vi "Main.vi"(8 "Error In":errorcluster, 11 "Simulate hardware?":bool) -> (0 "Error Out":errorcluster={"status"=FALSE, "code"=1073676294, "source"="VISA Read in Monochromator.lvlib:ReadWrite.vi->Monochromator.lvlib:move.vi:1990001->Monochromator.lvlib:moveBothMonos.vi->Monochromator.lvlib:Main.vi"})   [LabVIEW 2017, in "Monochromator.lvlib"]
uses:
  Monochromator.lvlib
  Controls/Commands [enum].ctl
  Controls/Params.ctl
  Controls/Type.ctl
  Controls/GratingValues.ctl
  Controls/Grating.ctl
  PTI/Controls/Params.ctl
  Controls/VISA parameters.ctl
  Custom Oriel drivers/Controls/Params.ctl
  C:/Project Work/icl-optical-software-rewrite/Optical Software Code Simplified/Modules/Monochromator/Cornerstone.dll
  Cornerstone.dll
  Events/Controls/Action Refs [enum].ctl
  PTI/PTI.lvlib
  System Control/Main controller.lvlib
  Events/Events.lvlib
  File IO/File IO.lvlib
  Custom Oriel drivers/Oriel (custom drivers).lvlib
  Serial comms/Serial comms.lvlib
panel:
  out "Monochromator out":T1={"Type"=enum."PTI", "Wavelength (nm)"=600.0, "Grating, gr/mm"=enum."1200", "Grating mode"=enum."Unknown", "Spectrum mode"={"Spectrum mode?"=FALSE, "Start wavelength (nm)"=0.0, "End wavelength (nm)"=0.0, "Wavelength step (nm)"=0.0, "Wavelength array"=[], "array index"=0}, "PTI"={"Delay before read (ms)"=300, "Mono 1"={"Timeout (ms)"=1000, "Resource Name"="COM5", "Baud Rate"=9600, "Data Bits"=8, "Parity"=0, "Stop Bits"=10, "Flow Control"=0}, "Mono 2"={"Timeout (ms)"=1000, "Resource Name"="COM6", "Baud Rate"=9600, "Data Bits"=8, "Parity"=0, "Stop Bits"=10, "Flow Control"=0}, "Two PTI Monochromators?"=FALSE}, "Oriel (custom)"={"reference"=refnum}, "Force wavelength confirmation (PTI)?"=FALSE} {"PTI"."Mono 2"."Flow Control" items=["1.0"=10, "1.5"=15, "2.0"=20]; "PTI"."Mono 2"."Stop Bits" items=["None", "Odd", "Even", "Mark", "Space"]; "PTI"."Mono 2"."Parity" items=["None", "Odd", "Even", "Mark", "Space"]; "PTI"."Mono 1"."Flow Control" items=["1.0"=10, "1.5"=15, "2.0"=20]; "PTI"."Mono 1"."Stop Bits" items=["None", "Odd", "Even", "Mark", "Space"]; "PTI"."Mono 1"."Parity" items=["None", "Odd", "Even", "Mark", "Space"]}
  out "Test":bool=TRUE
  in  "Monochromator":T1={"Type"=enum."PTI", "Wavelength (nm)"=600.0, "Grating, gr/mm"=enum."1200", "Grating mode"=enum."Unknown", "Spectrum mode"={"Spectrum mode?"=FALSE, "Start wavelength (nm)"=0.0, "End wavelength (nm)"=0.0, "Wavelength step (nm)"=0.0, "Wavelength array"=[], "array index"=0}, "PTI"={"Delay before read (ms)"=300, "Mono 1"={"Timeout (ms)"=1000, "Resource Name"="COM5", "Baud Rate"=9600, "Data Bits"=8, "Parity"=0, "Stop Bits"=10, "Flow Control"=0}, "Mono 2"={"Timeout (ms)"=1000, "Resource Name"="COM6", "Baud Rate"=9600, "Data Bits"=8, "Parity"=0, "Stop Bits"=10, "Flow Control"=0}, "Two PTI Monochromators?"=FALSE}, "Oriel (custom)"={"reference"=refnum}, "Force wavelength confirmation (PTI)?"=TRUE} {"PTI"."Mono 2"."Flow Control" items=["1.0"=10, "1.5"=15, "2.0"=20]; "PTI"."Mono 2"."Stop Bits" items=["None", "Odd", "Even", "Mark", "Space"]; "PTI"."Mono 2"."Parity" items=["None", "Odd", "Even", "Mark", "Space"]; "PTI"."Mono 1"."Flow Control" items=["1.0"=10, "1.5"=15, "2.0"=20]; "PTI"."Mono 1"."Stop Bits" items=["None", "Odd", "Even", "Mark", "Space"]; "PTI"."Mono 1"."Parity" items=["None", "Odd", "Even", "Mark", "Space"]}
  in  "Stop Button":bool
  in  "move to wavelength":dbl=200.0
  in  "State":T8
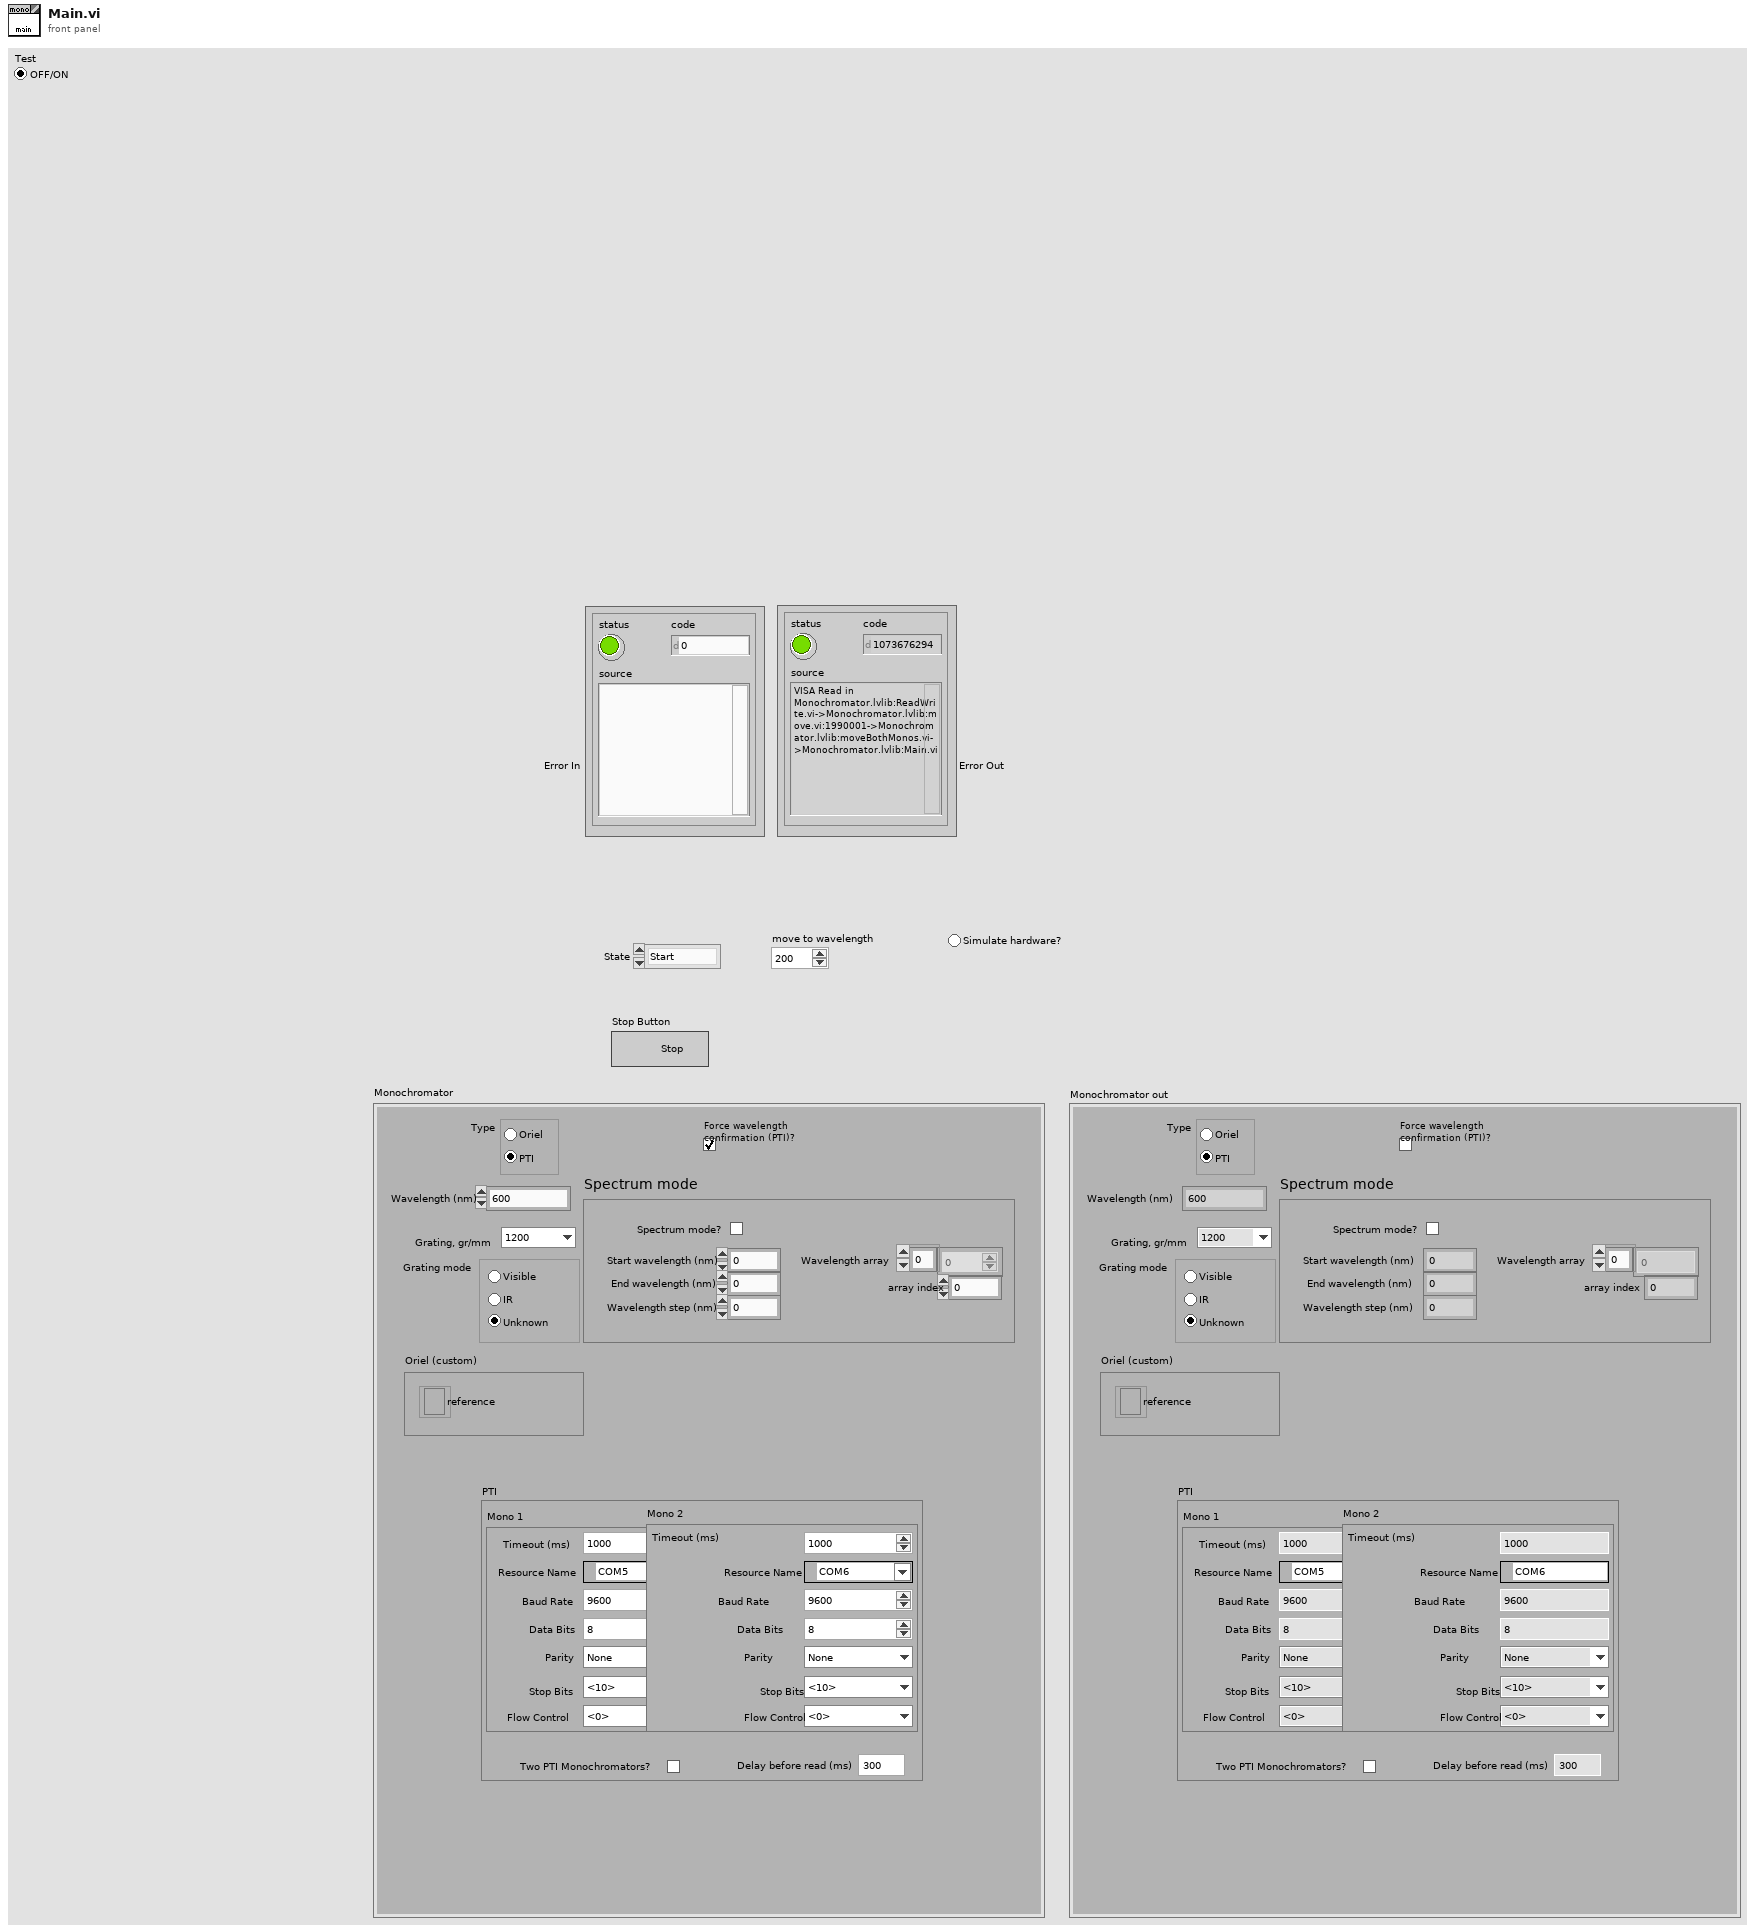
[diagram p1: front panel]
types:
  T1 = typedef "Monochromator.lvlib/Params.ctl" = cluster{"Type":T2, "Wavelength (nm)":dbl, "Grating, gr/mm":T3, "Grating mode":T4, "Spectrum mode":cluster{"Spectrum mode?":bool, "Start wavelength (nm)":dbl, "End wavelength (nm)":dbl, "Wavelength step (nm)":dbl, "Wavelength array":dbl[], "array index":u32}, "PTI":T5, "Oriel (custom)":T7, "Force wavelength confirmation (PTI)?":bool}
  T2 = typedef "Monochromator.lvlib/Type.ctl" = enum32{"Oriel", "PTI"}
  T3 = typedef "Monochromator.lvlib/GratingValues.ctl" = enum16{"2400", "1800", "1200", "600", "300", "150"}
  T4 = typedef "Monochromator.lvlib/Grating.ctl" = enum32{"Unknown", "Visible", "IR"}
  T5 = typedef "Monochromator.lvlib/PTI.lvlib/Params.ctl" = cluster{"Delay before read (ms)":u32, "Mono 1":T6, "Mono 2":T6, "Two PTI Monochromators?":bool}
  T6 = typedef "Serial comms.lvlib/VISA parameters.ctl" = cluster{"Timeout (ms)":u32, "Resource Name":refnum<visa-resource-name>, "Baud Rate":u32, "Data Bits":u16, "Parity":u16, "Stop Bits":u16, "Flow Control":u16}
  T7 = typedef "Monochromator.lvlib/Oriel (custom drivers).lvlib/Params.ctl" = cluster{"reference":refnum<k24>}
  T8 = typedef "Monochromator.lvlib/Commands [enum].ctl" = enum16{"Start", "Spectrum setup", "Spectrum move", "Monochromator Setup", "Move", "GetPosition", "Stop", "Send data"}
  T9 = enum32{"Bad", "Idle", "Run top level", "Running"}
  T10 = typedef "Events.lvlib/Action Refs [enum].ctl" = enum16{"Init", "Ref", "Kill"}
  T11 = typedef "Events.lvlib/Refs [cluster].ctl" = cluster{"Exit":refnum<user-event>, "Controller":refnum<user-event>, "System Error":refnum<user-event>, "UI":refnum<user-event>, "Example Module":refnum<user-event>, "Shutter":refnum<user-event>, "Monochromator":refnum<user-event>, "DAQ":refnum<user-event>, "Scope":refnum<user-event>, "Processing":refnum<user-event>, "File IO":refnum<user-event>, "Colour wheel":refnum<user-event>}
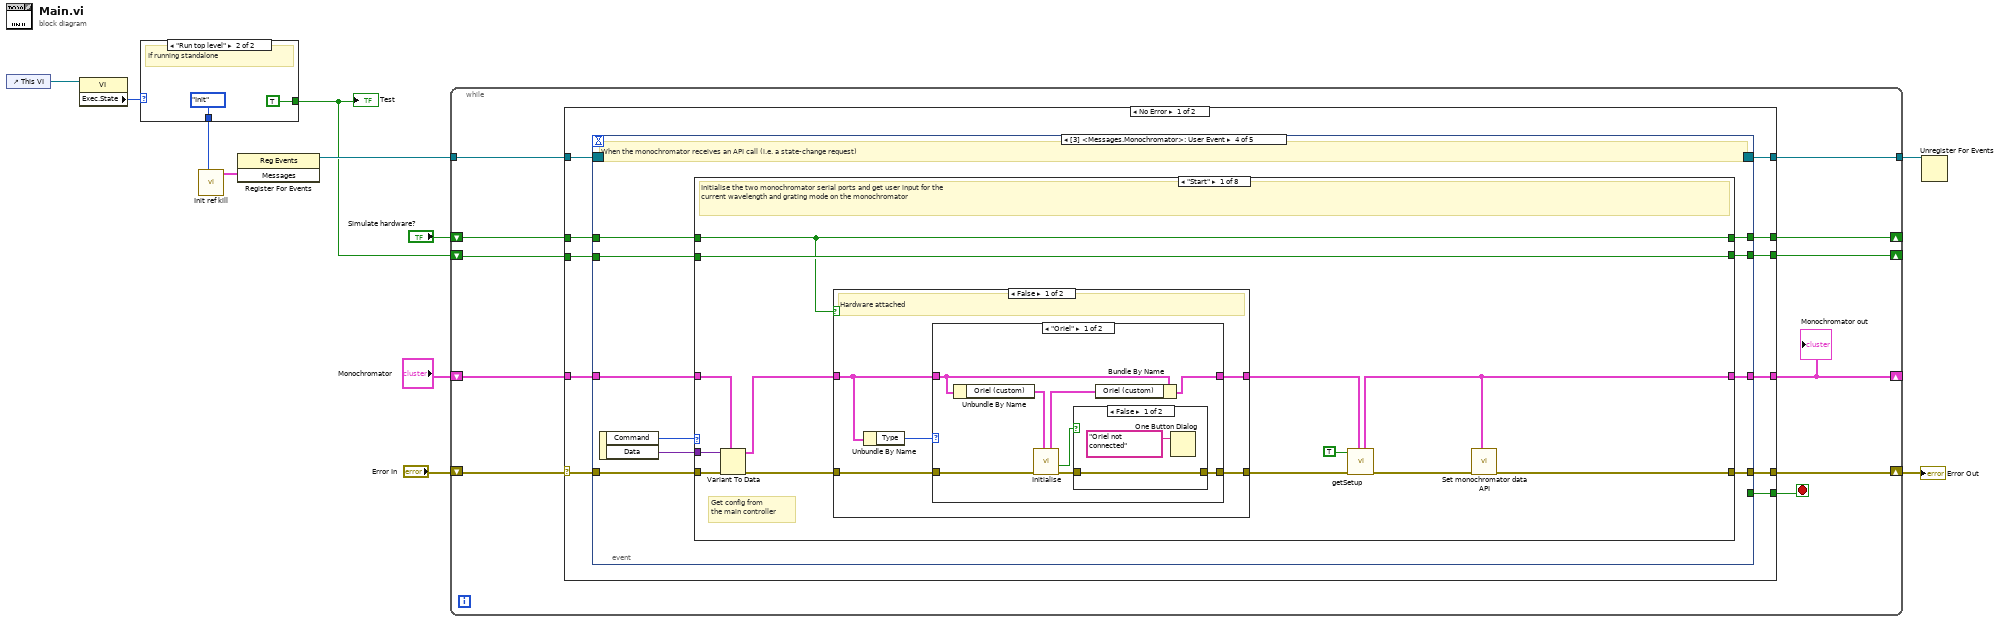
[diagram p0: block diagram]
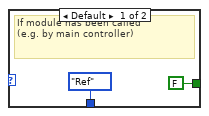
[diagram p2: hidden frame]
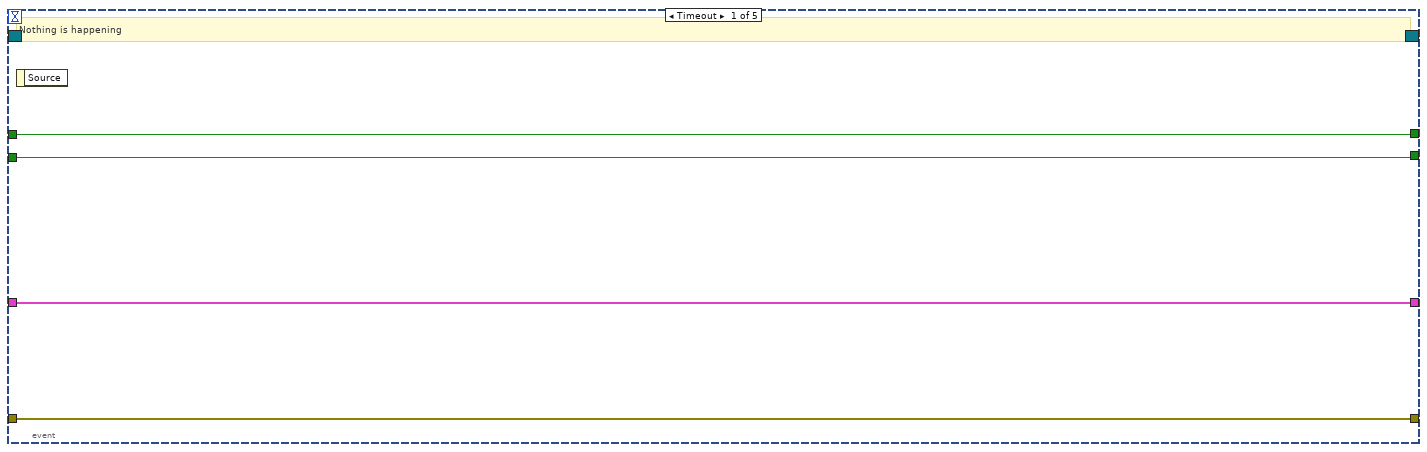
[diagram p3: hidden frame]
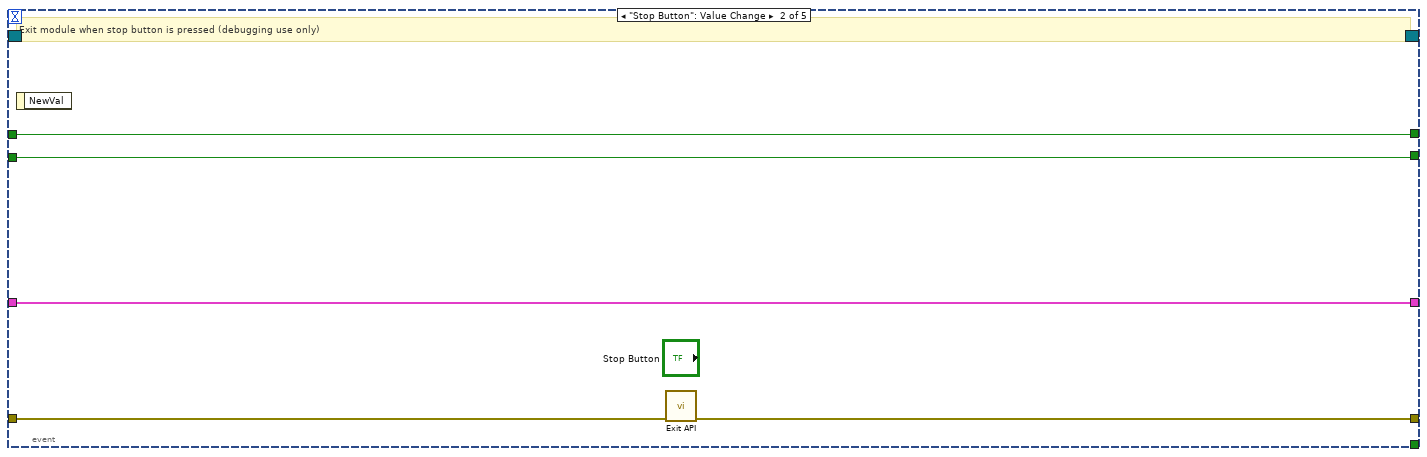
[diagram p4: hidden frame]
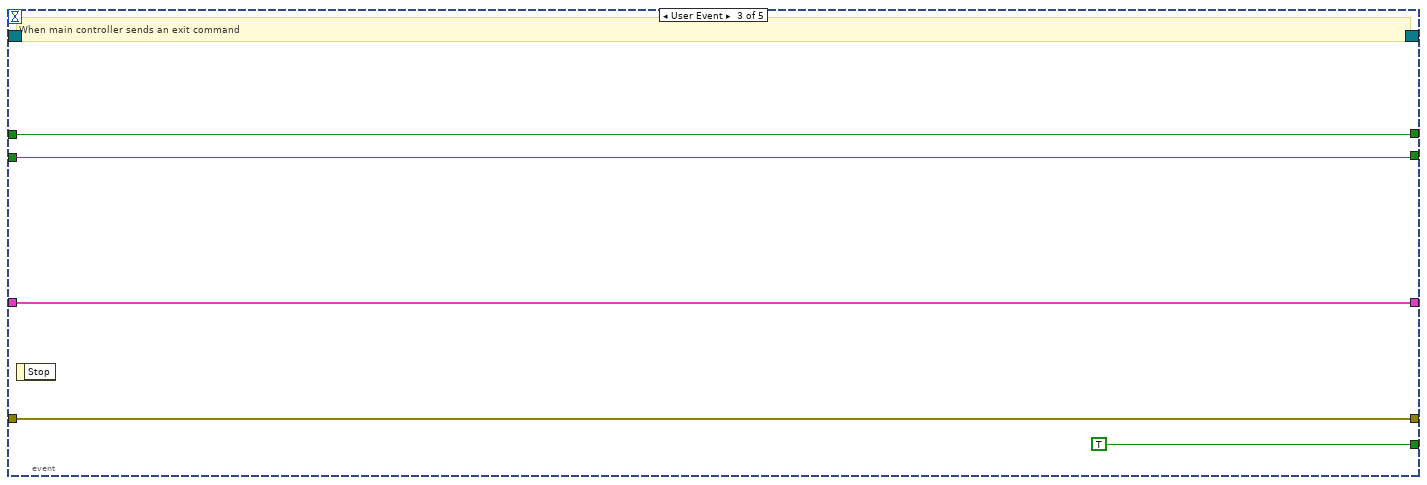
[diagram p5: hidden frame]
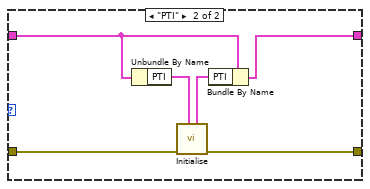
[diagram p7: hidden frame]
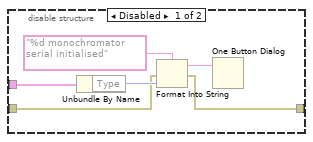
[diagram p9: hidden frame]
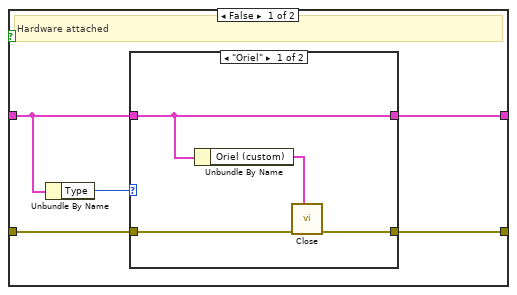
[diagram p11: hidden frame]
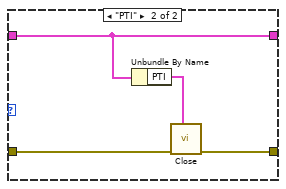
[diagram p12: hidden frame]
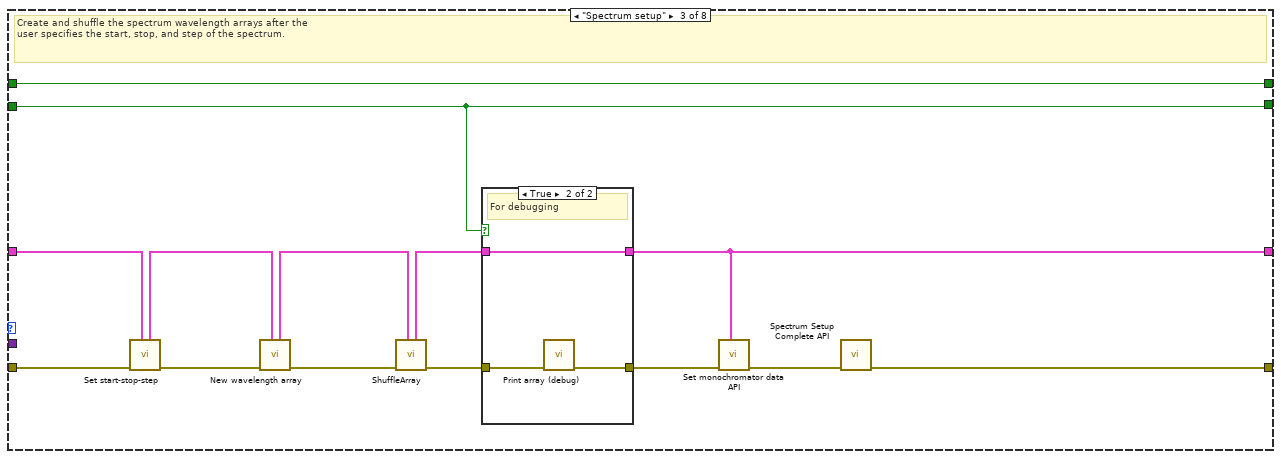
[diagram p13: hidden frame]
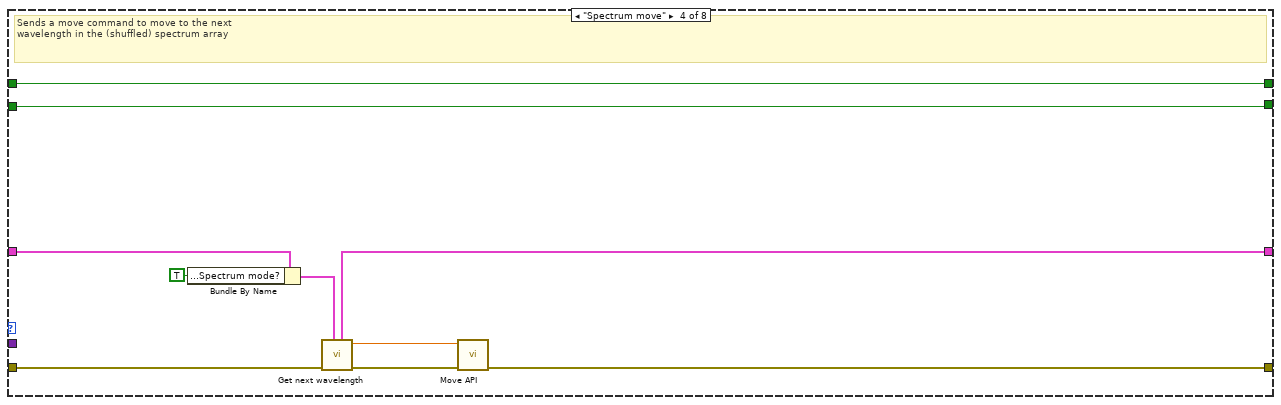
[diagram p15: hidden frame]
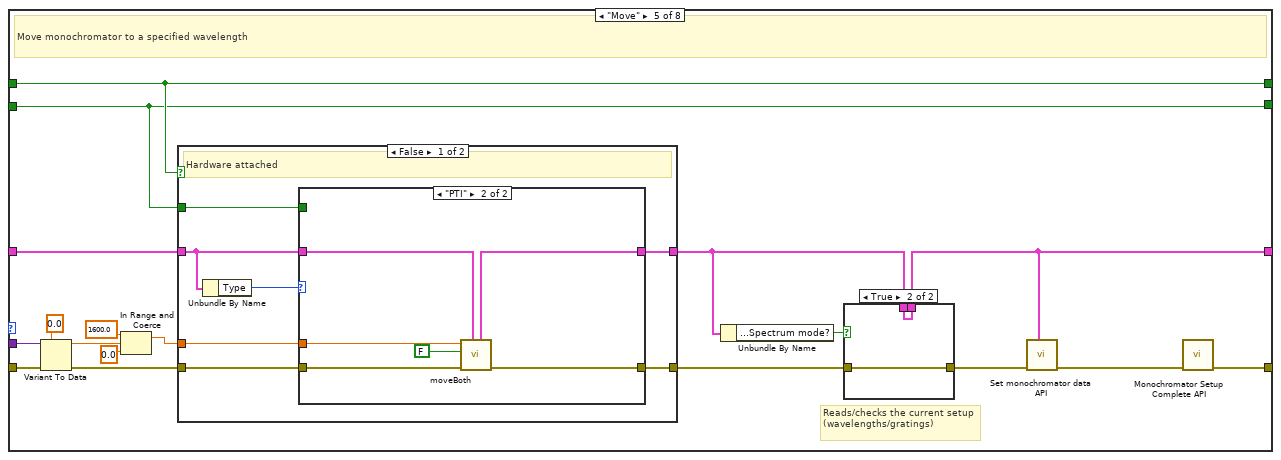
[diagram p16: hidden frame]
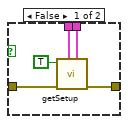
[diagram p17: hidden frame]
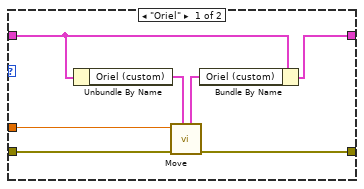
[diagram p18: hidden frame]
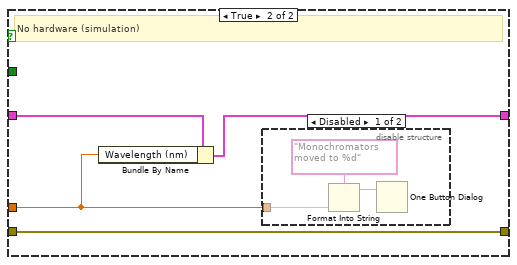
[diagram p19: hidden frame]
diagram:
  n1 = control-ref of="This VI"() -> (w6:refnum<vi>)
  n2 = property class="VI"(reference=w6) -> ("Exec.State"=w5:T9)  [unwired: 1 in, 2 out]
  n3 = case shown="\"Run top level\"" w5 {
    tunnel: [Action_Refs_[enum]."Ref" ("Action") Action_Refs_[enum]."Init" ("Action")] -> w4
    tunnel: [FALSE TRUE] -> w2
    frame Default {
      # "If module has been called\n(e.g. by main controller)"
    }
    frame "Run top level" {
      # "If running standalone"
    }
  }
  "Test" <- w2
  n4 = call "Init ref kill.vi"("Action"=w4) -> ("Messages"=w7:T11)  [unwired: 9 in, 1 out]
  n5 = register-events(w7) -> (reference out=w3:refnum<event-registration>)  [unwired: 2 in, 1 out]
  n6 = while {
    tunnel: [w25] -> w11
    shift-right: [w22] -> w9
    shift-left: "Error In" -> [w16]
    shift-right: [w23] -> _
    shift-left: "Monochromator" -> [w24]
    tunnel: w3 -> [w21]
    shift-right: [w19] -> _
    shift-left: "Simulate hardware?" -> [w20]
    shift-right: [w18] -> _
    shift-left: w2 -> [w17]
    stop <- w26 stop-if-true
    n7 = case shown="No Error" w16 {
      selector: w16 -> [w27 w306]
      tunnel: [w37 _] -> w26
      tunnel: [w36 w307] -> w25
      tunnel: w24 -> [w35 w310]
      tunnel: [w34 w310] -> w23
      tunnel: [w33 w304] -> w22
      tunnel: w21 -> [w32 w307]
      tunnel: w20 -> [w31 w309]
      tunnel: [w30 w309] -> w19
      tunnel: [w29 w308] -> w18
      tunnel: w17 -> [w28 w308]
      frame No Error {
        n8 = event shown="[3] <Messages.Monochromator>: User Event" {
          selector: w32 -> [_ _ _ _ _]
          dyn-events: [_ _ _ _ _] -> w36
          timeout: _ -> [_ _ _ _ _]
          tunnel: [_ _ TRUE _ _] -> w37
          tunnel: w27 -> [w40 w46 w50 w59 w283]
          tunnel: [w40 w45 w50 w58 w282] -> w33
          tunnel: w35 -> [w41 w42 w47 w56 w281]
          tunnel: [w41 w42 w47 w57 w280] -> w34
          tunnel: [w38 w43 w48 w55 w278] -> w30
          tunnel: w31 -> [w38 w43 w48 w54 w278]
          tunnel: [w39 w44 w49 w53 w279] -> w29
          tunnel: w28 -> [w39 w44 w49 w52 w279]
          event Timeout {
            # "Nothing is happening"
            n9 = event-data() -> ()  [unwired: 1 in, 1 out]
          }
          event "Stop Button": Value Change {
            # "Exit module when stop button is pressed (debugging use only)"
            n10 = event-data() -> ()  [unwired: 1 in, 1 out]
            n11 = call "Exit API.vi"("Error In"=w46) -> ("Error Out"=w45:errorcluster)  [unwired: 10 in]
          }
          event User Event {
            # "When main controller sends an exit command"
            n12 = event-data() -> ()  [unwired: 1 in, 1 out]
          }
          event User Event {
            # "When the monochromator receives an API call (i.e. a state-change request)"
            n13 = event-data() -> ("Command"=w61:T8, "Data"=w60:variant)  [unwired: 1 in]
            n14 = case shown="\"Start\"" w61 {
              tunnel: w60 -> [w71 _ _ _ w174 w225 _ _]
              tunnel: w59 -> [w73 w111 w137 w156 w172 w223 w262 w277]
              tunnel: [w65 w107 w131 w150 w162 w215 w260 w276] -> w58
              tunnel: w56 -> [w70 w112 w139 w149 w170 w212 w259 w275]
              tunnel: [w63 w110 w128 w153 w159 w210 w261 w275] -> w57
              tunnel: [w67 w109 w134 w151 w168 w220 w265 w273] -> w55
              tunnel: w54 -> [w67 w109 w134 w151 w168 w220 w265 w273]
              tunnel: w52 -> [w68 w108 w133 w152 w167 w219 w264 w274]
              tunnel: [w68 w108 w133 w152 w167 w219 w264 w274] -> w53
              frame "Start" {
                # "Get config from\nthe main controller"
                # "Initialise the two monochromator serial ports and get user input for the \ncurrent wavelength and grating mode on the monochromator"
                n15 = Variant To Data(error in=w73, type=w70, Variant=w71) -> (data=w69:T1, error out=w72:errorcluster)
                n16 = case shown="False" w67 {
                  tunnel: [w77 w97] -> w66
                  tunnel: [w79 w98] -> w74
                  tunnel: w72 -> [w78 w99]
                  tunnel: w69 -> [w76 w97]
                  frame False {
                    # "Hardware attached"
                    n17 = Unbundle By Name(w76) -> ("Type"=w75:T2)
                    n18 = case shown="\"Oriel\"" w75 {
                      tunnel: [w80 w96] -> w79
                      tunnel: w78 -> [w87 w95]
                      tunnel: [w85 w92] -> w77
                      tunnel: w76 -> [w86 w91]
                      frame "Oriel" {
                        n19 = Unbundle By Name(w86) -> ("Oriel (custom)"=w84:T7)
                        n20 = call "Initialise.vi"("Oriel (custom drivers)"=w84, "error in (no error)"=w87) -> ("error out"=w81:errorcluster, "Mono Connected?"=w82:bool, "Oriel (custom drivers) out"=w83:T7)  [unwired: 7 in]
                        n21 = case shown="False" w82 {
                          tunnel: w81 -> [w88 w90]
                          tunnel: [w88 w90] -> w80
                          frame False {
                            n22 = One Button Dialog(message="Oriel not connected") -> ()  [unwired: 1 in, 1 out]
                          }
                          frame True {
                          }
                        }
                        n23 = Bundle By Name(cluster=w86, "Oriel (custom)"=w83) -> (w85:T1)
                      }
                      frame "PTI" {
                        n24 = Unbundle By Name(w91) -> ("PTI"=w94:T5)
                        n25 = call "Initialise.vi"("PTI in"=w94, "error in (no error)"=w95) -> ("error out"=w96:errorcluster, "PTI out"=w93:T5)  [unwired: 8 in]
                        n26 = Bundle By Name(cluster=w91, "PTI"=w93) -> (w92:T1)
                      }
                    }
                  }
                  frame True {
                    # "No hardware (simulation)"
                    n27 = disable-structure shown="Enabled" {
                      disable-tunnel: w99 -> [w102 w106]
                      disable-tunnel: [w101 w106] -> w98
                      disable-tunnel: w97 -> [w100 _]
                      frame Disabled {
                        n28 = Unbundle By Name(w100) -> ("Type"=w105:T2)
                        n29 = Format Into String(format string="%d monochromator serial initialised" ("initial string"), error in=w102, w105) -> (resulting string=w104:string, error out=w101:errorcluster)  [unwired: 1 in]
                        n30 = One Button Dialog(message=w104) -> ()  [unwired: 1 in, 1 out]
                      }
                      frame Enabled {
                      }
                    }
                  }
                }
                n31 = call "getSetup.vi"("Monochromator in"=w66, "error in (no error)"=w74, "Enable wavelength input? (T)"=TRUE ("Disable wavelength input (F)")) -> ("error out"=w64:errorcluster, "Monochromator out"=w63:T1)  [unwired: 7 in]
                n32 = call "Set monochromator data API.vi"("Monochromator"=w63, "Error In"=w64) -> ("Error Out"=w65:errorcluster)  [unwired: 9 in]
              }
              frame "Stop" {
                # "Close the two monochromator serial ports"
                n33 = case shown="True" w109 {
                  tunnel: w112 -> [w113 w126]
                  tunnel: w111 -> [w117 w127]
                  tunnel: [w116 w127] -> w107
                  tunnel: [w115 w126] -> w110
                  frame False {
                    # "Hardware attached"
                    n34 = Unbundle By Name(w113) -> ("Type"=w114:T2)
                    n35 = case shown="\"Oriel\"" w114 {
                      tunnel: [w121 w125] -> w116
                      tunnel: [w119 w123] -> w115
                      tunnel: w113 -> [w119 w123]
                      tunnel: w117 -> [w120 w122]
                      frame "Oriel" {
                        n36 = Unbundle By Name(w119) -> ("Oriel (custom)"=w118:T7)
                        n37 = call "Close.vi"("Monochromator in"=w118, "error in (no error)"=w120) -> ("error out"=w121:errorcluster)  [unwired: 9 in]
                      }
                      frame "PTI" {
                        n38 = Unbundle By Name(w123) -> ("PTI"=w124:T5)
                        n39 = call "Close.vi"("PTI"=w124, "error in (no error)"=w122) -> ("error out"=w125:errorcluster)  [unwired: 9 in]
                      }
                    }
                  }
                  frame True {
                    # "No hardware (simulation)"
                  }
                }
              }
              frame "Spectrum setup" {
                # "Create and shuffle the spectrum wavelength arrays after the \nuser specifies the start, stop, and step of the spectrum."
                n40 = call "Set start-stop-step.vi"("Monochromator in"=w139, "error in (no error)"=w137) -> ("error out"=w136:errorcluster, "Monochromator"=w138:T1)  [unwired: 8 in]
                n41 = call "New wavelength array.vi"("Monochromator in"=w138, "Error In"=w136) -> ("Error Out"=w140:errorcluster, "Monochromator out"=w141:T1)  [unwired: 8 in]
                n42 = call "ShuffleArray.vi"("Monochromator in"=w141, "Error In"=w140) -> ("Error Out"=w135:errorcluster, "Monochromator out"=w132:T1)  [unwired: 8 in]
                n43 = case shown="True" w133 {
                  tunnel: w135 -> [w143 w146]
                  tunnel: [w143 w145] -> w130
                  tunnel: w132 -> [w142 w144]
                  tunnel: [w142 w144] -> w128
                  frame False {
                  }
                  frame True {
                    # "For debugging"
                    n44 = call "Print array (debug).vi"("Error In"=w146) -> ("Error Out"=w145:errorcluster)  [unwired: 10 in]
                  }
                }
                n45 = call "Set monochromator data API.vi"("Monochromator"=w128, "Error In"=w130) -> ("Error Out"=w129:errorcluster)  [unwired: 9 in]
                n46 = call "Spectrum Setup Complete API.vi"("Error In"=w129) -> ("Error Out"=w131:errorcluster)  [unwired: 10 in]
              }
              frame "Spectrum move" {
                # "Sends a move command to move to the next \nwavelength in the (shuffled) spectrum array"
                n47 = Bundle By Name(cluster=w149, "Spectrum mode.Spectrum mode?"=TRUE) -> (w148:T1)
                n48 = call "Get next wavelength.vi"("Monochromator in"=w148, "Error In"=w156) -> ("Error Out"=w155:errorcluster, "destination wavelength (nm)"=w154:dbl, "Monochromator out"=w153:T1)  [unwired: 7 in]
                n49 = call "Move API.vi"("Error In"=w155, "wavelength"=w154) -> ("Error Out"=w150:errorcluster)  [unwired: 9 in]
              }
              frame "Move" {
                # "Reads/checks the current setup (wavelengths/gratings)"
                # "Move monochromator to a specified wavelength"
                n50 = Variant To Data(error in=w172, type=0.0, Variant=w174) -> (data=w171:dbl, error out=w164:errorcluster)
                n51 = In Range and Coerce(upper limit=1600.0, x=w171, lower limit=0.0) -> (coerced(x)=w169:dbl)  [unwired: 1 out]
                n52 = case shown="False" w168 {
                  tunnel: [w187 w203] -> w160
                  tunnel: [w188 w205] -> w163
                  tunnel: w164 -> [w186 w205]
                  tunnel: w170 -> [w184 w204]
                  tunnel: w169 -> [w185 w202]
                  tunnel: w167 -> [w182 _]
                  frame False {
                    # "Hardware attached"
                    n53 = Unbundle By Name(w184) -> ("Type"=w183:T2)
                    n54 = case shown="\"PTI\"" w183 {
                      tunnel: [w195 w201] -> w188
                      tunnel: [w193 w200] -> w187
                      tunnel: w186 -> [w194 w199]
                      tunnel: w184 -> [w192 w197]
                      tunnel: w185 -> [w191 w198]
                      tunnel: w182 -> [_ _]
                      frame "Oriel" {
                        n55 = Unbundle By Name(w192) -> ("Oriel (custom)"=w189:T7)
                        n56 = call "Move.vi"("Oriel (custom drivers) in"=w189, "error in (no error)"=w194, "Wavelength"=w191) -> ("error out"=w195:errorcluster, "Oriel (custom drivers) out"=w190:T7)  [unwired: 6 in, 1 out]
                        n57 = Bundle By Name(cluster=w192, "Oriel (custom)"=w190) -> (w193:T1)
                      }
                      frame "PTI" {
                        n58 = call "moveBoth.vi"("Monochromator in"=w197, "error in (no error)"=w199, "Debug messages?"=FALSE, "wavelength"=w198) -> ("error out"=w201:errorcluster, "Monochromator out"=w200:T1)  [unwired: 6 in]
                      }
                    }
                  }
                  frame True {
                    # "No hardware (simulation)"
                    n59 = Bundle By Name(cluster=w204, "Wavelength (nm)"=w202) -> (w203:T1)
                    n60 = disable-structure shown="Disabled" {
                      disable-tunnel: w202 -> [w206 _]
                      frame Disabled {
                        n61 = Format Into String(format string="Monochromators moved to %d" ("message"), w206) -> (resulting string=w208:string)  [unwired: 2 in, 1 out]
                        n62 = One Button Dialog(message=w208) -> ()  [unwired: 1 in, 1 out]
                      }
                      frame Enabled {
                      }
                    }
                  }
                }
                n63 = Unbundle By Name(w160) -> ("Spectrum mode.Spectrum mode?"=w157:bool)
                n64 = case shown="True" w157 {
                  tunnel: [w178 w180] -> w158
                  tunnel: w163 -> [w177 w180]
                  tunnel: w160 -> [w176 w181]
                  tunnel: [w175 w181] -> w159
                  frame False {
                    n65 = call "getSetup.vi"("Monochromator in"=w176, "error in (no error)"=w177, "Enable wavelength input? (T)"=TRUE ("Disable wavelength input (F)")) -> ("error out"=w178:errorcluster, "Monochromator out"=w175:T1)  [unwired: 7 in]
                  }
                  frame True {
                  }
                }
                n66 = call "Set monochromator data API.vi"("Monochromator"=w159, "Error In"=w158) -> ("Error Out"=w161:errorcluster)  [unwired: 9 in]
                n67 = call "Monochromator Setup Complete API.vi"("Error In"=w161) -> ("Error Out"=w162:errorcluster)  [unwired: 10 in]
              }
              frame "Monochromator Setup" {
                # "Move monochromator to a specified wavelength"
                n68 = Variant To Data(error in=w223, type=0.0, Variant=w225) -> (data=w222:dbl, error out=w216:errorcluster)
                n69 = Bundle By Name(cluster=w212, "Spectrum mode.Spectrum mode?"=FALSE) -> (w211:T1)
                n70 = In Range and Coerce(upper limit=1600.0, x=w222, lower limit=0.0) -> (coerced(x)=w221:dbl)  [unwired: 1 out]
                n71 = case shown="False" w220 {
                  tunnel: [w231 w253] -> w210
                  tunnel: [w232 w257] -> w209
                  tunnel: w216 -> [w230 w257]
                  tunnel: w211 -> [w228 w254]
                  tunnel: w221 -> [w229 w252]
                  tunnel: w219 -> [w226 _]
                  frame False {
                    # "Hardware attached"
                    n72 = Unbundle By Name(w228) -> ("Type"=w227:T2)
                    n73 = case shown="\"Oriel\"" w227 {
                      tunnel: [w233 w251] -> w232
                      tunnel: [w239 w250] -> w231
                      tunnel: w230 -> [w240 w249]
                      tunnel: w228 -> [w238 w247]
                      tunnel: w229 -> [w235 w248]
                      tunnel: w226 -> [_ w246]
                      frame "Oriel" {
                        n74 = Unbundle By Name(w238) -> ("Oriel (custom)"=w236:T7)
                        n75 = call "Move.vi"("Oriel (custom drivers) in"=w236, "error in (no error)"=w240, "Wavelength"=w235) -> ("error out"=w233:errorcluster, "Wavelength Set"=w234:bool, "Oriel (custom drivers) out"=w237:T7)  [unwired: 6 in]
                        n76 = case shown="True" w234 {
                          tunnel: [w241 w245] -> w239
                          tunnel: w238 -> [w241 w244]
                          tunnel: w237 -> [_ w243]
                          tunnel: w235 -> [_ w242]
                          frame False {
                          }
                          frame True {
                            n77 = Bundle By Name(cluster=w244, "Oriel (custom)"=w243, "Wavelength (nm)"=w242) -> (w245:T1)
                          }
                        }
                      }
                      frame "PTI" {
                        n78 = call "moveBoth.vi"("Monochromator in"=w247, "error in (no error)"=w249, "Debug messages?"=w246, "wavelength"=w248) -> ("error out"=w251:errorcluster, "Monochromator out"=w250:T1)  [unwired: 6 in]
                      }
                    }
                  }
                  frame True {
                    # "No hardware (simulation)"
                    n79 = Bundle By Name(cluster=w254, "Wavelength (nm)"=w252) -> (w253:T1)
                    n80 = Format Into String(format string="Monochromators moved to %d" ("message"), w252) -> (resulting string=w256:string)  [unwired: 2 in, 1 out]
                    n81 = One Button Dialog(message=w256) -> ()  [unwired: 1 in, 1 out]
                  }
                }
                n82 = call "Set monochromator data API.vi"("Monochromator"=w210, "Error In"=w209) -> ("Error Out"=w214:errorcluster)  [unwired: 9 in]
                n83 = call "Monochromator Setup Complete API.vi"("Error In"=w214) -> ("Error Out"=w215:errorcluster)  [unwired: 10 in]
              }
              frame "GetPosition" {
                # "Update the main controller"
                n84 = Unbundle By Name(w259) -> ("Spectrum mode.Spectrum mode?"=w258:bool)
                n85 = case shown="False" w258 {
                  tunnel: [w269 w271] -> w263
                  tunnel: w262 -> [w268 w271]
                  tunnel: w259 -> [w267 w272]
                  tunnel: [w266 w272] -> w261
                  frame False {
                    # "Reads/checks the current setup (wavelengths/gratings)"
                    n86 = call "getSetup.vi"("Monochromator in"=w267, "error in (no error)"=w268, "Enable wavelength input? (T)"=TRUE ("Disable wavelength input (F)")) -> ("error out"=w269:errorcluster, "Monochromator out"=w266:T1)  [unwired: 7 in]
                  }
                  frame True {
                  }
                }
                n87 = call "Send params API.vi"("Error In"=w263) -> ("Error Out"=w260:errorcluster)  [unwired: 10 in]
              }
              frame "Send data" {
                # "Send a message to the UI module to update the display \nwith the new monochromator parameters"
                n88 = call "Set monochromator data API.vi"("Monochromator"=w275, "Error In"=w277) -> ("Error Out"=w276:errorcluster)  [unwired: 9 in]
              }
            }
          }
          event Value Change {
            # "Used for standalone running/testing of the module"
            n89 = event-data() -> ("NewVal"=w284:T8)  [unwired: 1 in]
            n90 = case shown="\"Start\", Default" w284 {
              tunnel: w283 -> [w287 w290 w293 w297 w300 w303]
              tunnel: [w286 w289 w292 w296 w299 w302] -> w282
              tunnel: w281 -> [w285 w288 w291 w294 w298 w301]
              tunnel: [w285 w288 w291 w294 w298 w301] -> w280
              frame "Start", Default {
                n91 = call "Start API.vi"("Monochromator"=w285, "Error In"=w287) -> ("Error Out"=w286:errorcluster)  [unwired: 9 in]
              }
              frame "Spectrum setup" {
                n92 = call "Spectrum Setup API.vi"("Error In"=w290) -> ("Error Out"=w289:errorcluster)  [unwired: 10 in]
              }
              frame "Spectrum move" {
                n93 = call "Spectrum Move API.vi"("Error In"=w293) -> ("Error Out"=w292:errorcluster)  [unwired: 10 in]
              }
              frame "Move" {
                n94 = call "Move API.vi"("Error In"=w297, "wavelength"="move to wavelength") -> ("Error Out"=w296:errorcluster)  [unwired: 9 in]
              }
              frame "Stop" {
                n95 = call "Stop API.vi"("Error In"=w300) -> ("Error Out"=w299:errorcluster)  [unwired: 10 in]
              }
              frame "Send data" {
                n96 = call "Send params API.vi"("Error In"=w303) -> ("Error Out"=w302:errorcluster)  [unwired: 10 in]
              }
            }
          }
        }
      }
      frame Error {
        n97 = local read "Test"() -> (w305:bool)
        n98 = case shown="False" w305 {
          tunnel: [w312 _] -> w304
          tunnel: w306 -> [w311 w317]
          frame False {
            n99 = case shown="Error" w311 {
              selector: w311 -> [w313 w315]
              tunnel: [w313 w316] -> w312
              frame No Error {
              }
              frame Error {
                n100 = call "Send Error API.vi"("Error Cluster"=w315) -> ("Error Out"=w314:errorcluster)  [unwired: 10 in]
                n101 = call "Log error API.vi"("Error In"=w314) -> ("Error Out"=w316:errorcluster)  [unwired: 10 in]
              }
            }
          }
          frame True {
            n102 = call <vilib>:"Simple Error Handler.vi"("error in (no error)"=w317) -> ()  [unwired: 4 in, 5 out]
          }
        }
      }
    }
    "Monochromator out" <- w23
  }
  "Error Out" <- w9
  n103 = Unregister For Events(event registration refnum=w11) -> ()  [unwired: 1 in, 1 out]
